vi "Mod_OFDM_Seed_Initialization.vi"(0 "Data Sources":i8[](array[numeric]), 1 "Register Initial State":u32, 2 "Data Source.Reset to Initial State":T1(ring), 9 "Seed IN":i32, 11 "error in (no error)":errorcluster, 13 "Data Source":u16) -> (4 "Data Sources":i8[](array[numeric]), 10 "Seed OUT":i32, 15 "error out":errorcluster)   [LabVIEW 2010]
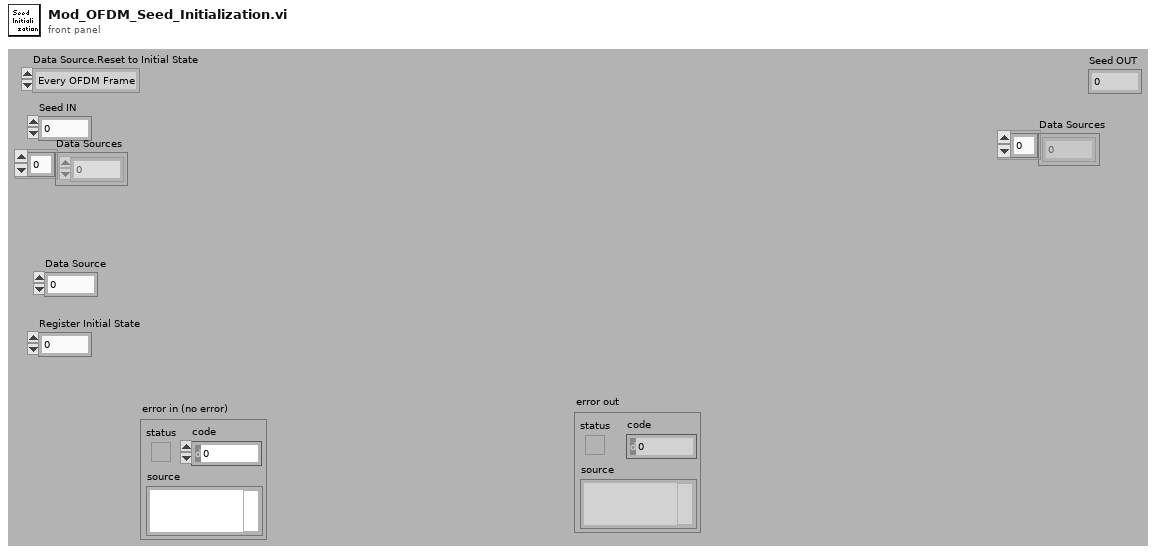
[diagram p1: front panel]
types:
  T1 = enum16{"Every OFDM Frame", "Every OFDM Symbol", "Every Sub Carrier"}
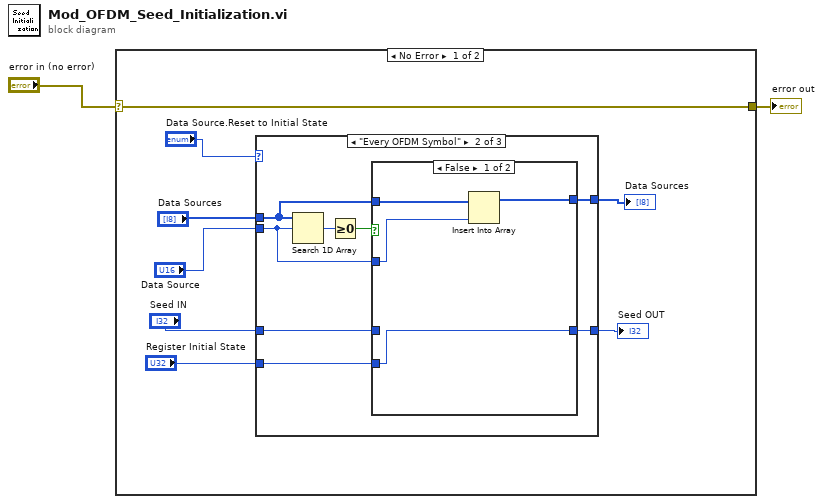
[diagram p0: block diagram]
diagram:
  n1 = case shown="No Error" "error in (no error)" {
    selector: "error in (no error)" -> [w4 w29]
    tunnel: [w4 w29] -> w1
    frame No Error {
      n2 = case shown="\"Every OFDM Symbol\"" "Data Source.Reset to Initial State" {
        tunnel: "Seed IN" -> [_ w18 w28]
        tunnel: [w11 w17 w28] -> w8
        tunnel: "Data Sources" -> [w12 w16 w27]
        tunnel: "Data Source" -> [_ w15 _]
        tunnel: [w12 w14 w27] -> w5
        tunnel: "Register Initial State" -> [w11 w13 _]
        frame "Every Sub Carrier", Default {
        }
        frame "Every OFDM Symbol" {
          n3 = Search 1D Array(1D array=w16, element=w15) -> (index of element=w20:i32)  [unwired: 1 in]
          n4 = Greater Or Equal To 0?(x=w20) -> (x >= 0?=w19:bool)
          n5 = case shown="False" w19 {
            tunnel: w18 -> [_ w26]
            tunnel: [w21 w26] -> w17
            tunnel: w16 -> [w24 w25]
            tunnel: w15 -> [w23 _]
            tunnel: [w22 w25] -> w14
            tunnel: w13 -> [w21 _]
            frame False {
              n6 = Insert Into Array(array=w24, new element=w23) -> (w22:i8[])  [unwired: 1 in]
            }
            frame True {
            }
          }
        }
        frame "Every OFDM Frame" {
        }
      }
      "Seed OUT" <- w8
      "Data Sources" <- w5
    }
    frame Error {
    }
  }
  "error out" <- w1
